vi "testCustomFailureMessage.vi"() -> ()   [LabVIEW 2019, in "AssertionTest.lvlib" / "AssertRefnum.lvlib"]
uses:
  Constraint/IsRefnum/Create.vi
  Constraint/IsRefnum/IsRefnum.lvclass
  AssertRefnum.lvlib
  Assertion/Assertion.lvlib
panel:
  out "error out":errorcluster
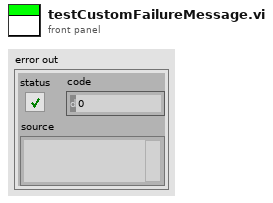
[diagram p1: front panel]
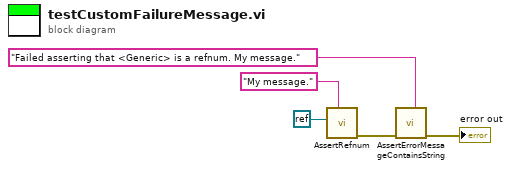
[diagram p0: block diagram]
diagram:
  n1 = call "AssertRefnum.vi"("Message (\"\")"="My message." ("Message (\"\")"), "Refnum"=refnum<k0> refnum) -> ("error out"=w5:errorcluster)  [unwired: 9 in]
  n2 = call "AssertErrorMessageContainsString.vi"("Expected"="Failed asserting that <Generic> is a refnum. My message.", "error in (no error)"=w5) -> ("error out"=→"error out":errorcluster)  [unwired: 9 in]
